vi "calcInc.vi"(1 "no. steps":i32, 2 "init pos (mm)":dbl, 3 "fin pos (mm)":dbl) -> (0 "inc (mm)":dbl)   [LabVIEW 2015]
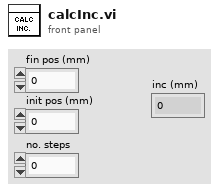
[diagram p1: front panel]
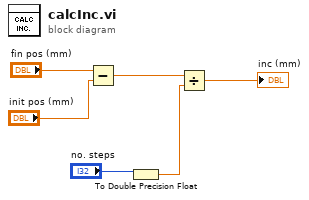
[diagram p0: block diagram]
diagram:
  n1 = Subtract(x="fin pos (mm)", y="init pos (mm)") -> (x-y=w1:dbl)
  n2 = To Double Precision Float(number="no. steps") -> (double precision float=w3:dbl)
  n3 = Divide(x=w1, y=w3) -> (x/y=→"inc (mm)":dbl)
